vi "Clear pretomo IMAQ.vi"(8 "error in (no error)":errorcluster, 11 "Tomo in":refnum<class "Tomo.lvclass">) -> (0 "error out":errorcluster, 3 "Tomo out":refnum<class "Tomo.lvclass">)   [LabVIEW 2012, in "Tomo.lvclass"]
uses:
  Tomo.lvclass
  Tomo.lvclass/Tomo.ctl
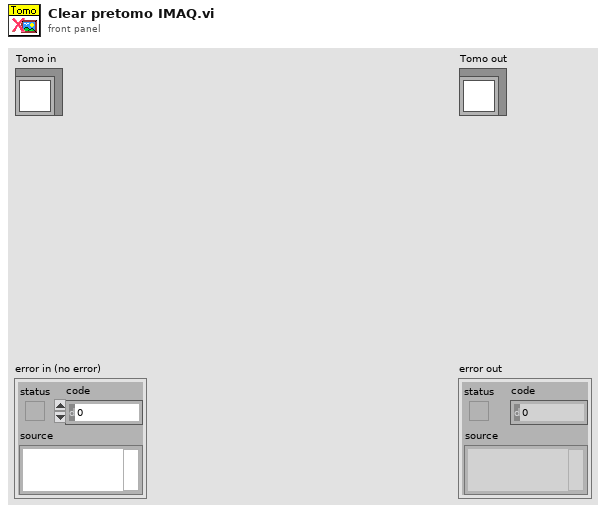
[diagram p1: front panel]
types:
  T1 = typedef "IMAQ Image.ctl" = refnum<image>
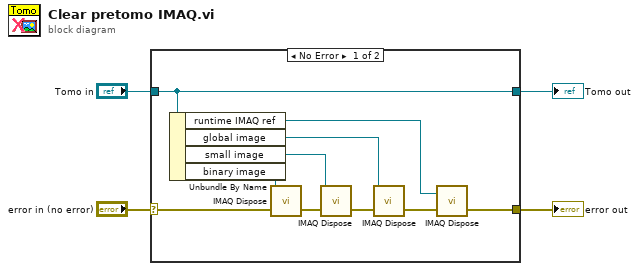
[diagram p0: block diagram]
diagram:
  n1 = case shown="No Error" "error in (no error)" {
    selector: "error in (no error)" -> [w11 w16]
    tunnel: [w6 w16] -> w3
    tunnel: [w14 w15] -> w1
    tunnel: "Tomo in" -> [w14 w15]
    frame No Error {
      n2 = Unbundle By Name(w14) -> ("runtime IMAQ ref"=w5:T1, "global image"=w8:T1, "small image"=w9:T1, "binary image"=w10:T1)
      n3 = call "IMAQ Dispose"("Image"=w10, "error in (no error)"=w11) -> ("error out"=w13:errorcluster)  [unwired: 4 in]
      n4 = call "IMAQ Dispose"("Image"=w9, "error in (no error)"=w13) -> ("error out"=w12:errorcluster)  [unwired: 4 in]
      n5 = call "IMAQ Dispose"("Image"=w8, "error in (no error)"=w12) -> ("error out"=w7:errorcluster)  [unwired: 4 in]
      n6 = call "IMAQ Dispose"("Image"=w5, "error in (no error)"=w7) -> ("error out"=w6:errorcluster)  [unwired: 4 in]
    }
    frame Error {
    }
  }
  "error out" <- w3
  "Tomo out" <- w1
